vi "IrInitializeBootstrap.vi"(8 "error in (no error)":errorcluster) -> (0 "error out":errorcluster, 2 "ProcessName":string, 3 "Qbus out":refnum<class "Qbus.lvclass">)   [LabVIEW 2017]
uses:
  <vilib>/addons/Qbus/Qbus.lvclass
  <vilib>/addons/InsightCM/Devices/Shared/Common/ServerComm/ServerComm.lvlib
  <vilib>/addons/TimerProcess/TimerProcess.lvlib
  <vilib>/addons/TraceLogger/TraceLogger.lvlib
  <vilib>/addons/InsightCM/Utilities/GlobalConfiguration/GlobalConfiguration.lvlib
  <vilib>/addons/SystemInfoProcess/SystemInfoProcess.lvlib
  <vilib>/addons/BlinkProcess/BlinkProcess.lvlib
  <vilib>/addons/InsightCM/Devices/Shared/Common/Controller/Controller.lvlib
  <vilib>/addons/InsightCM/Devices/Shared/Ir/IrManageCameras/IrManageCameras.lvlib
  <vilib>/addons/InsightCM/Devices/Shared/Ir/IrAcquisition/IrAcquisition.lvlib
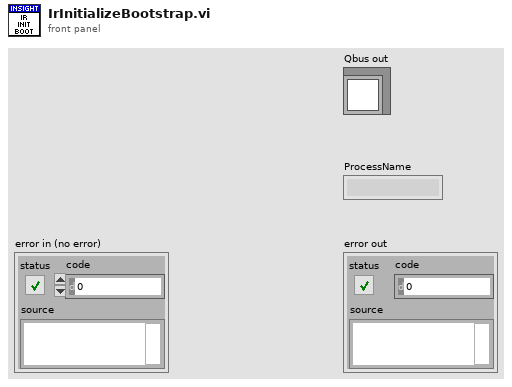
[diagram p1: front panel]
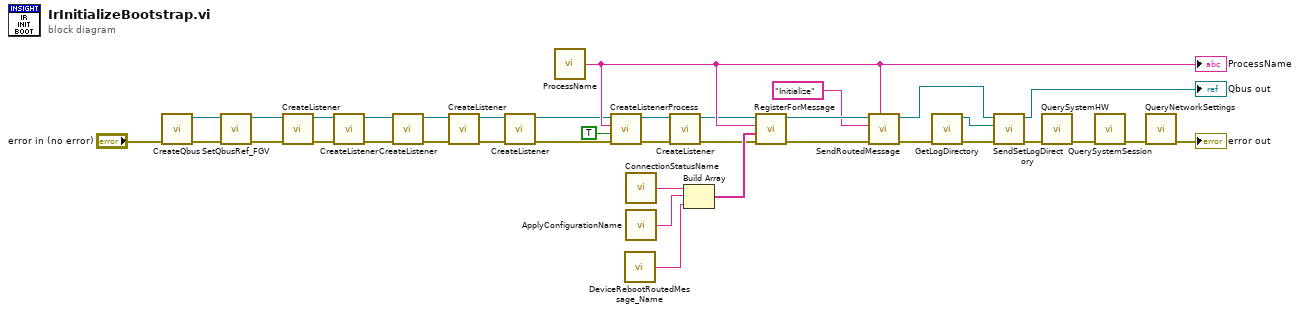
[diagram p0: block diagram]
diagram:
  n1 = call <vilib>:"CreateQbus.vi"("error in (no error)"="error in (no error)") -> ("error out"=w15:errorcluster, "Qbus"=w16:refnum<class "Qbus.lvclass">)  [unwired: 9 in]
  n2 = call <vilib>:"SetQbusRef_FGV.vi"("error in (no error)"=w15, "Qbus in"=w16) -> ("error out"=w13:errorcluster, "Qbus out"=w14:refnum<class "Qbus.lvclass">)  [unwired: 8 in]
  n3 = call <vilib>:"CreateListener.vi"("error in (no error)"=w13, "Qbus in"=w14) -> ("error out"=w37:errorcluster, "Qbus out"=w36:refnum<class "Qbus.lvclass">)  [unwired: 8 in]
  n4 = call <vilib>:"CreateListener.vi"("error in (no error)"=w37, "qbus in"=w36) -> ("error out"=w31:errorcluster, "qbus out"=w30:refnum<class "Qbus.lvclass">)  [unwired: 8 in]
  n5 = call <vilib>:"CreateListener.vi"("error in (no error)"=w31, "qbus in"=w30) -> ("error out"=w3:errorcluster, "qbus out"=w6:refnum<class "Qbus.lvclass">)  [unwired: 8 in]
  n6 = call <vilib>:"CreateListener.vi"("error in (no error)"=w3, "Qbus in"=w6) -> ("error out"=w2:errorcluster, "Qbus out"=w5:refnum<class "Qbus.lvclass">)  [unwired: 8 in]
  n7 = call <vilib>:"CreateListener.vi"("error in (no error)"=w2, "Qbus in"=w5) -> ("error out"=w1:errorcluster, "Qbus out"=w4:refnum<class "Qbus.lvclass">)  [unwired: 8 in]
  n8 = call <vilib>:"ProcessName.vi"() -> ("ProcessName"=w12:string)  [unwired: 5 in]
  "ProcessName" <- w12
  n9 = call <vilib>:"CreateListenerProcess.vi"("error in (no error)"=w1, "master"=TRUE ("Master"), "process name"=w12, "Qbus in"=w4) -> ("error in (no error)"=w8:errorcluster, "Qbus out"=w7:refnum<class "Qbus.lvclass">)  [unwired: 6 in]
  n10 = call <vilib>:"DeviceRebootRoutedMessage_Name.vi"() -> ("MessageName"=w11:string)  [unwired: 5 in]
  n11 = call <vilib>:"ConnectionStatusName.vi"() -> ("message name"=w35:string)  [unwired: 5 in]
  n12 = call <vilib>:"ApplyConfigurationName.vi"() -> ("message name"=w17:string)  [unwired: 5 in]
  n13 = call <vilib>:"CreateListener.vi"("error in (no error)"=w8, "Qbus in"=w7) -> ("error out"=w9:errorcluster, "Qbus out"=w10:refnum<class "Qbus.lvclass">)  [unwired: 8 in]
  n14 = Build Array(w35, w17, w11) -> (w34:string[])
  n15 = call <vilib>:"RegisterForMessage.vi"("error in (no error)"=w9, "message names"=w34, "process name"=w12, "Qbus in"=w10) -> ("error in (no error)"=w28:errorcluster, "Qbus out"=w29:refnum<class "Qbus.lvclass">)  [unwired: 6 in]
  n16 = call <vilib>:"SendRoutedMessage.vi"("listener process"=w12, "error in (no error)"=w28, "message name"="Initialize", "Qbus in"=w29) -> ("error in (no error)"=w24:errorcluster, "Qbus out"=w19:refnum<class "Qbus.lvclass">)  [unwired: 6 in]
  n17 = call <vilib>:"GetLogDirectory.vi"("error in (no error)"=w24) -> ("error out"=w25:errorcluster, "log dir"=w26:path)  [unwired: 9 in]
  n18 = call <vilib>:"SendSetLogDirectory.vi"("error in (no error)"=w25, "log directory"=w26, "qbus in"=w19) -> ("error out"=w23:errorcluster, "qbus out"=→"Qbus out":refnum<class "Qbus.lvclass">)  [unwired: 7 in]
  n19 = call <vilib>:"QuerySystemHW.vi"("error in (no error)"=w23) -> ("error out"=w22:errorcluster)  [unwired: 10 in]
  n20 = call <vilib>:"QuerySystemSession.vi"("error in (no error)"=w22) -> ("error out"=w21:errorcluster)  [unwired: 10 in]
  n21 = call <vilib>:"QueryNetworkSettings.vi"("error in (no error)"=w21) -> ("error out"=→"error out":errorcluster)  [unwired: 10 in]
